vi "LoadGlobeSettings.vi"(8 "error in (no error)":errorcluster, 11 "Tree DVR in":refnum<data-value>) -> (0 "error out":errorcluster, 3 "Global Settings":T1)   [LabVIEW 2014]
uses:
  <vilib>/MDSplus/Classes/Tree_Class/Tree.lvclass
  Controls/Global Settings/GlobalSettings.ctl
  Controls/Global Settings/InitialBackgroundValues.ctl
  Controls/Global Settings/GasPuffing.ctl
  Controls/Global Settings/PSUVoltages.ctl
  Controls/Global Settings/ScopeDetails.ctl
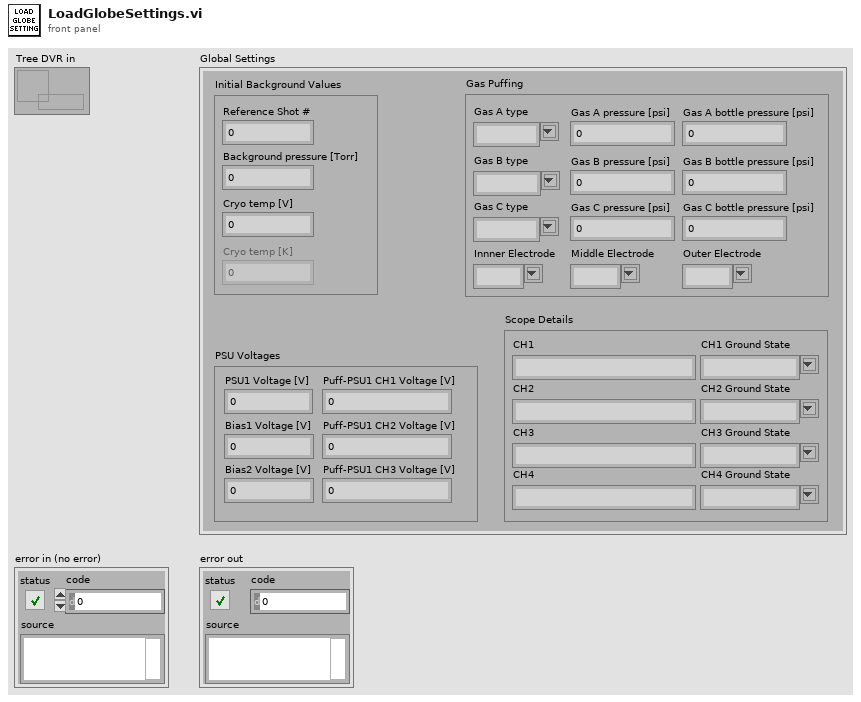
[diagram p1: front panel]
types:
  T1 = typedef "GlobalSettings.ctl" = cluster{"Initial Background Values":T2, "Gas Puffing":T3, "PSU Voltages":T4, "Scope Details":T5}
  T2 = typedef "InitialBackgroundValues.ctl" = cluster{"Reference Shot #":dbl, "Background pressure [Torr]":dbl, "Cryo temp [V]":dbl, "Cryo temp [K]":dbl}
  T3 = typedef "GasPuffing.ctl" = cluster{"Gas A type":string, "Gas B type":string, "Gas C type":string, "Gas A pressure [psi]":dbl, "Gas B pressure [psi]":dbl, "Gas C pressure [psi]":dbl, "Innner Electrode":string, "Middle Electrode":string, "Outer Electrode":string, "Gas A bottle pressure [psi]":dbl, "Gas B bottle pressure [psi]":dbl, "Gas C bottle pressure [psi]":dbl}
  T4 = typedef "PSUVoltages.ctl" = cluster{"Bias1 Voltage [V]":dbl, "Bias2 Voltage [V]":dbl, "PSU1 Voltage [V]":dbl, "Puff-PSU1 CH1 Voltage [V]":dbl, "Puff-PSU1 CH2 Voltage [V]":dbl, "Puff-PSU1 CH3 Voltage [V]":dbl}
  T5 = typedef "ScopeDetails.ctl" = cluster{"CH1":string, "CH2":string, "CH3":string, "CH4":string, "CH1 Ground State":string, "CH2 Ground State":string, "CH3 Ground State":string, "CH4 Ground State":string}
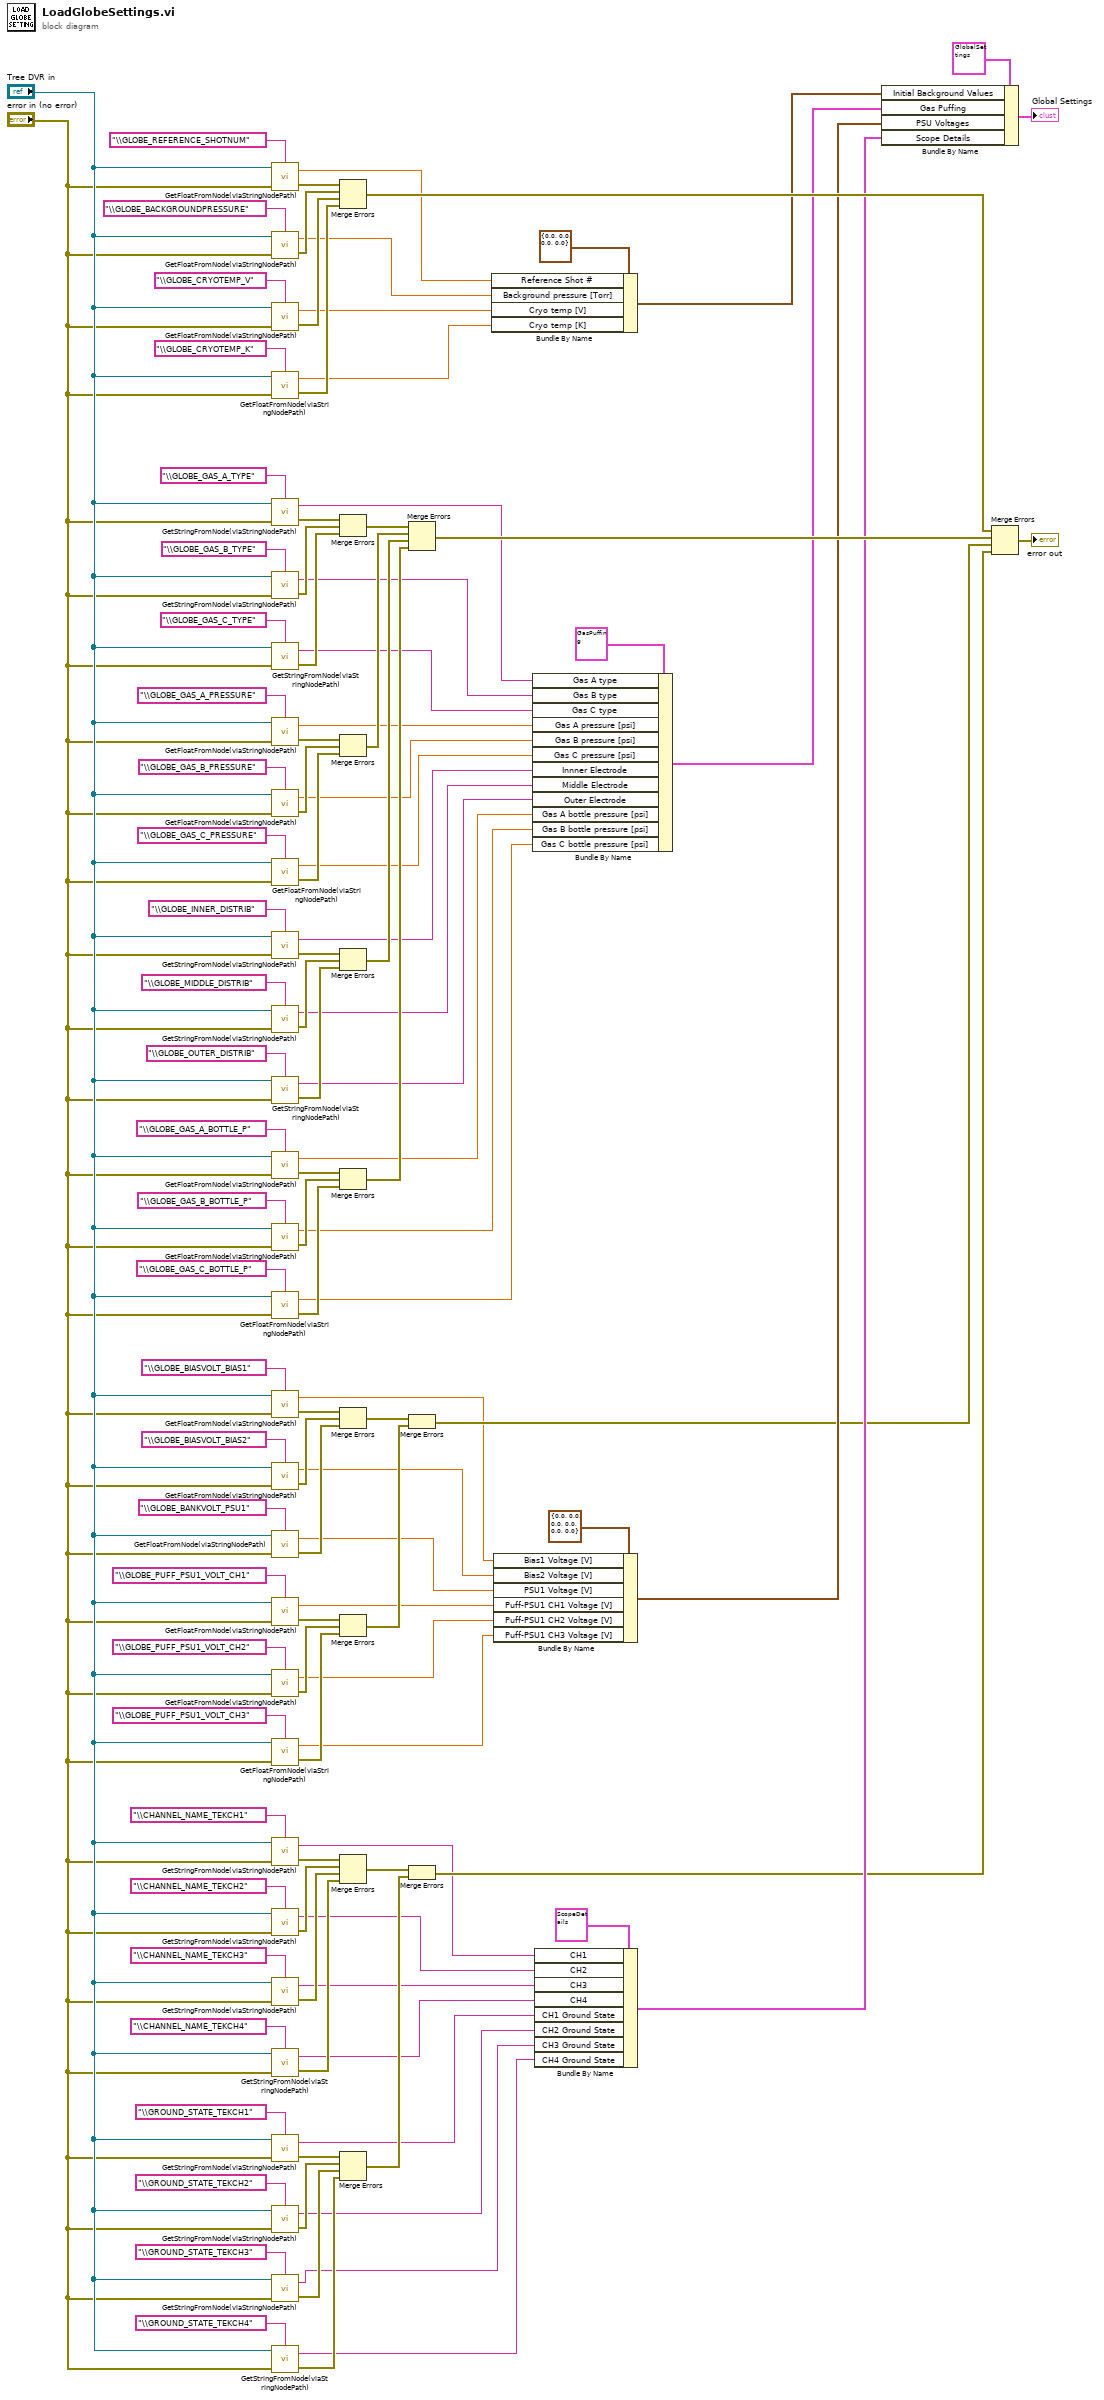
[diagram p0: block diagram]
diagram:
  n1 = call "GetFloatFromNode(viaStringNodePath).vi"("Path"="\\GLOBE_REFERENCE_SHOTNUM", "error in"="error in (no error)", "Tree DVR in"="Tree DVR in") -> ("error out"=w60:errorcluster, "Float64"=w4:dbl)  [unwired: 1 in]
  n2 = call "GetFloatFromNode(viaStringNodePath).vi"("Path"="\\GLOBE_BACKGROUNDPRESSURE", "error in"="error in (no error)", "Tree DVR in"="Tree DVR in") -> ("error out"=w59:errorcluster, "Float64"=w3:dbl)  [unwired: 1 in]
  n3 = call "GetFloatFromNode(viaStringNodePath).vi"("Path"="\\GLOBE_CRYOTEMP_V", "error in"="error in (no error)", "Tree DVR in"="Tree DVR in") -> ("error out"=w58:errorcluster, "Float64"=w2:dbl)  [unwired: 1 in]
  n4 = call "GetFloatFromNode(viaStringNodePath).vi"("Path"="\\GLOBE_CRYOTEMP_K", "error in"="error in (no error)", "Tree DVR in"="Tree DVR in") -> ("error out"=w57:errorcluster, "Float64"=w1:dbl)  [unwired: 1 in]
  n5 = call "GetStringFromNode(viaStringNodePath).vi"("Path"="\\GLOBE_GAS_A_TYPE", "error in"="error in (no error)", "Tree DVR in"="Tree DVR in") -> ("error out"=w56:errorcluster, "String out"=w16:string)  [unwired: 1 in]
  n6 = call "GetStringFromNode(viaStringNodePath).vi"("Path"="\\GLOBE_GAS_B_TYPE", "error in"="error in (no error)", "Tree DVR in"="Tree DVR in") -> ("error out"=w55:errorcluster, "String out"=w15:string)  [unwired: 1 in]
  n7 = call "GetStringFromNode(viaStringNodePath).vi"("Path"="\\GLOBE_GAS_C_TYPE", "error in"="error in (no error)", "Tree DVR in"="Tree DVR in") -> ("error out"=w54:errorcluster, "String out"=w14:string)  [unwired: 1 in]
  n8 = call "GetFloatFromNode(viaStringNodePath).vi"("Path"="\\GLOBE_GAS_A_PRESSURE", "error in"="error in (no error)", "Tree DVR in"="Tree DVR in") -> ("error out"=w53:errorcluster, "Float64"=w13:dbl)  [unwired: 1 in]
  n9 = call "GetFloatFromNode(viaStringNodePath).vi"("Path"="\\GLOBE_GAS_B_PRESSURE", "error in"="error in (no error)", "Tree DVR in"="Tree DVR in") -> ("error out"=w52:errorcluster, "Float64"=w12:dbl)  [unwired: 1 in]
  n10 = call "GetFloatFromNode(viaStringNodePath).vi"("Path"="\\GLOBE_GAS_C_PRESSURE", "error in"="error in (no error)", "Tree DVR in"="Tree DVR in") -> ("error out"=w51:errorcluster, "Float64"=w11:dbl)  [unwired: 1 in]
  n11 = call "GetStringFromNode(viaStringNodePath).vi"("Path"="\\GLOBE_INNER_DISTRIB", "error in"="error in (no error)", "Tree DVR in"="Tree DVR in") -> ("error out"=w50:errorcluster, "String out"=w10:string)  [unwired: 1 in]
  n12 = call "GetStringFromNode(viaStringNodePath).vi"("Path"="\\GLOBE_MIDDLE_DISTRIB", "error in"="error in (no error)", "Tree DVR in"="Tree DVR in") -> ("error out"=w49:errorcluster, "String out"=w9:string)  [unwired: 1 in]
  n13 = call "GetStringFromNode(viaStringNodePath).vi"("Path"="\\GLOBE_OUTER_DISTRIB", "error in"="error in (no error)", "Tree DVR in"="Tree DVR in") -> ("error out"=w48:errorcluster, "String out"=w8:string)  [unwired: 1 in]
  n14 = call "GetFloatFromNode(viaStringNodePath).vi"("Path"="\\GLOBE_GAS_A_BOTTLE_P", "error in"="error in (no error)", "Tree DVR in"="Tree DVR in") -> ("error out"=w47:errorcluster, "Float64"=w7:dbl)  [unwired: 1 in]
  n15 = call "GetFloatFromNode(viaStringNodePath).vi"("Path"="\\GLOBE_GAS_B_BOTTLE_P", "error in"="error in (no error)", "Tree DVR in"="Tree DVR in") -> ("error out"=w46:errorcluster, "Float64"=w6:dbl)  [unwired: 1 in]
  n16 = call "GetFloatFromNode(viaStringNodePath).vi"("Path"="\\GLOBE_GAS_C_BOTTLE_P", "error in"="error in (no error)", "Tree DVR in"="Tree DVR in") -> ("error out"=w45:errorcluster, "Float64"=w5:dbl)  [unwired: 1 in]
  n17 = call "GetFloatFromNode(viaStringNodePath).vi"("Path"="\\GLOBE_BIASVOLT_BIAS1", "error in"="error in (no error)", "Tree DVR in"="Tree DVR in") -> ("error out"=w44:errorcluster, "Float64"=w22:dbl)  [unwired: 1 in]
  n18 = call "GetFloatFromNode(viaStringNodePath).vi"("Path"="\\GLOBE_BIASVOLT_BIAS2", "error in"="error in (no error)", "Tree DVR in"="Tree DVR in") -> ("error out"=w43:errorcluster, "Float64"=w21:dbl)  [unwired: 1 in]
  n19 = call "GetFloatFromNode(viaStringNodePath).vi"("Path"="\\GLOBE_BANKVOLT_PSU1", "error in"="error in (no error)", "Tree DVR in"="Tree DVR in") -> ("error out"=w42:errorcluster, "Float64"=w20:dbl)  [unwired: 1 in]
  n20 = call "GetFloatFromNode(viaStringNodePath).vi"("Path"="\\GLOBE_PUFF_PSU1_VOLT_CH1", "error in"="error in (no error)", "Tree DVR in"="Tree DVR in") -> ("error out"=w41:errorcluster, "Float64"=w19:dbl)  [unwired: 1 in]
  n21 = call "GetFloatFromNode(viaStringNodePath).vi"("Path"="\\GLOBE_PUFF_PSU1_VOLT_CH2", "error in"="error in (no error)", "Tree DVR in"="Tree DVR in") -> ("error out"=w40:errorcluster, "Float64"=w18:dbl)  [unwired: 1 in]
  n22 = call "GetFloatFromNode(viaStringNodePath).vi"("Path"="\\GLOBE_PUFF_PSU1_VOLT_CH3", "error in"="error in (no error)", "Tree DVR in"="Tree DVR in") -> ("error out"=w39:errorcluster, "Float64"=w17:dbl)  [unwired: 1 in]
  n23 = call "GetStringFromNode(viaStringNodePath).vi"("Path"="\\CHANNEL_NAME_TEKCH1", "error in"="error in (no error)", "Tree DVR in"="Tree DVR in") -> ("error out"=w38:errorcluster, "String out"=w30:string)  [unwired: 1 in]
  n24 = call "GetStringFromNode(viaStringNodePath).vi"("Path"="\\CHANNEL_NAME_TEKCH2", "error in"="error in (no error)", "Tree DVR in"="Tree DVR in") -> ("error out"=w37:errorcluster, "String out"=w29:string)  [unwired: 1 in]
  n25 = call "GetStringFromNode(viaStringNodePath).vi"("Path"="\\CHANNEL_NAME_TEKCH3", "error in"="error in (no error)", "Tree DVR in"="Tree DVR in") -> ("error out"=w36:errorcluster, "String out"=w28:string)  [unwired: 1 in]
  n26 = call "GetStringFromNode(viaStringNodePath).vi"("Path"="\\CHANNEL_NAME_TEKCH4", "error in"="error in (no error)", "Tree DVR in"="Tree DVR in") -> ("error out"=w35:errorcluster, "String out"=w27:string)  [unwired: 1 in]
  n27 = call "GetStringFromNode(viaStringNodePath).vi"("Path"="\\GROUND_STATE_TEKCH1", "error in"="error in (no error)", "Tree DVR in"="Tree DVR in") -> ("error out"=w34:errorcluster, "String out"=w26:string)  [unwired: 1 in]
  n28 = call "GetStringFromNode(viaStringNodePath).vi"("Path"="\\GROUND_STATE_TEKCH2", "error in"="error in (no error)", "Tree DVR in"="Tree DVR in") -> ("error out"=w33:errorcluster, "String out"=w25:string)  [unwired: 1 in]
  n29 = call "GetStringFromNode(viaStringNodePath).vi"("Path"="\\GROUND_STATE_TEKCH3", "error in"="error in (no error)", "Tree DVR in"="Tree DVR in") -> ("error out"=w32:errorcluster, "String out"=w24:string)  [unwired: 1 in]
  n30 = call "GetStringFromNode(viaStringNodePath).vi"("Path"="\\GROUND_STATE_TEKCH4", "error in"="error in (no error)", "Tree DVR in"="Tree DVR in") -> ("error out"=w31:errorcluster, "String out"=w23:string)  [unwired: 1 in]
  n31 = Merge Errors(w60, w59, w58, w57) -> (w78:errorcluster)
  n32 = Merge Errors(w56, w55, w54) -> (w77:errorcluster)
  n33 = Merge Errors(w53, w52, w51) -> (w76:errorcluster)
  n34 = Merge Errors(w50, w49, w48) -> (w75:errorcluster)
  n35 = Merge Errors(w47, w46, w45) -> (w74:errorcluster)
  n36 = Merge Errors(w44, w43, w42) -> (w68:errorcluster)
  n37 = Merge Errors(w41, w40, w39) -> (w67:errorcluster)
  n38 = Merge Errors(w38, w37, w36, w35) -> (w66:errorcluster)
  n39 = Merge Errors(w34, w33, w32, w31) -> (w65:errorcluster)
  n40 = Merge Errors(w77, w76, w75, w74) -> (w73:errorcluster)
  n41 = Merge Errors(w68, w67) -> (w64:errorcluster)
  n42 = Merge Errors(w66, w65) -> (w63:errorcluster)
  n43 = Bundle By Name(cluster=T2 {"Reference Shot #"=0.0, "Background pressure [Torr]"=0.0, "Cryo temp [V]"=0.0, "Cryo temp [K]"=0.0} ("Initial Background Values"), "Reference Shot #"=w4, "Background pressure [Torr]"=w3, "Cryo temp [V]"=w2, "Cryo temp [K]"=w1) -> (w72:T2)
  n44 = Bundle By Name(cluster=T4 {"Bias1 Voltage [V]"=0.0, "Bias2 Voltage [V]"=0.0, "PSU1 Voltage [V]"=0.0, "Puff-PSU1 CH1 Voltage [V]"=0.0, "Puff-PSU1 CH2 Voltage [V]"=0.0, "Puff-PSU1 CH3 Voltage [V]"=0.0} ("PSU Voltages"), "Bias1 Voltage [V]"=w22, "Bias2 Voltage [V]"=w21, "PSU1 Voltage [V]"=w20, "Puff-PSU1 CH1 Voltage [V]"=w19, "Puff-PSU1 CH2 Voltage [V]"=w18, "Puff-PSU1 CH3 Voltage [V]"=w17) -> (w70:T4)
  n45 = Bundle By Name(cluster=T3 {"Gas A type"="N", "Gas B type"="N", "Gas C type"="N", "Gas A pressure [psi]"=0.0, "Gas B pressure [psi]"=0.0, "Gas C pressure [psi]"=0.0, "Innner Electrode"="", "Middle Electrode"="", "Outer Electrode"="", "Gas A bottle pressure [psi]"=0.0, "Gas B bottle pressure [psi]"=0.0, "Gas C bottle pressure [psi]"=0.0} ("Gas Puffing"), "Gas A type"=w16, "Gas B type"=w15, "Gas C type"=w14, "Gas A pressure [psi]"=w13, "Gas B pressure [psi]"=w12, "Gas C pressure [psi]"=w11, "Innner Electrode"=w10, "Middle Electrode"=w9, "Outer Electrode"=w8, "Gas A bottle pressure [psi]"=w7, "Gas B bottle pressure [psi]"=w6, "Gas C bottle pressure [psi]"=w5) -> (w71:T3)
  n46 = Bundle By Name(cluster=T5 {"CH1"="", "CH2"="", "CH3"="", "CH4"="", "CH1 Ground State"="Grounded", "CH2 Ground State"="Grounded", "CH3 Ground State"="Grounded", "CH4 Ground State"="Grounded"} ("Scope Details"), "CH1"=w30, "CH2"=w29, "CH3"=w28, "CH4"=w27, "CH1 Ground State"=w26, "CH2 Ground State"=w25, "CH3 Ground State"=w24, "CH4 Ground State"=w23) -> (w69:T5)
  n47 = Bundle By Name(cluster=T1 {"Initial Background Values"={"Reference Shot #"=0.0, "Background pressure [Torr]"=0.0, "Cryo temp [V]"=0.0, "Cryo temp [K]"=0.0}, "Gas Puffing"={"Gas A type"="N", "Gas B type"="N", "Gas C type"="N", "Gas A pressure [psi]"=0.0, "Gas B pressure [psi]"=0.0, "Gas C pressure [psi]"=0.0, "Innner Electrode"="", "Middle Electrode"="", "Outer Electrode"="", "Gas A bottle pressure [psi]"=0.0, "Gas B bottle pressure [psi]"=0.0, "Gas C bottle pressure [psi]"=0.0}, "PSU Voltages"={"Bias1 Voltage [V]"=0.0, "Bias2 Voltage [V]"=0.0, "PSU1 Voltage [V]"=0.0, "Puff-PSU1 CH1 Voltage [V]"=0.0, "Puff-PSU1 CH2 Voltage [V]"=0.0, "Puff-PSU1 CH3 Voltage [V]"=0.0}, "Scope Details"={"CH1"="", "CH2"="", "CH3"="", "CH4"="", "CH1 Ground State"="Grounded", "CH2 Ground State"="Grounded", "CH3 Ground State"="Grounded", "CH4 Ground State"="Grounded"}} ("Global Settings"), "Initial Background Values"=w72, "Gas Puffing"=w71, "PSU Voltages"=w70, "Scope Details"=w69) -> (→"Global Settings":T1)
  n48 = Merge Errors(w78, w73, w64, w63) -> (→"error out":errorcluster)
